vi "firstImageInArray.vi"(1 "Array":T1[](array[typedef])) -> (0 "Image":T1)   [LabVIEW 2015]
uses:
  <vilib>/vision/Image Controls.llb/IMAQ Image.ctl
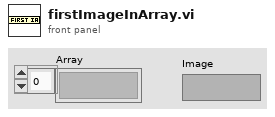
[diagram p1: front panel]
types:
  T1 = typedef "IMAQ Image.ctl" = refnum<image>
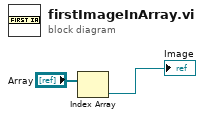
[diagram p0: block diagram]
diagram:
  n1 = Index Array(array="Array") -> (element=→"Image":T1)  [unwired: 1 in]
